vi "Data Type to I32.vi"(8 "error in (no error)":errorcluster, 11 "Data Type":refnum<class "Data Type.lvclass">) -> (0 "error out":errorcluster, 3 "I32 out":i32)   [LabVIEW 2017, in "I32.lvclass"]
uses:
  <vilib>/gpm_packages/@cs/data-type-serializer/source/I32/I32.lvclass
  <vilib>/gpm_packages/@cs/data-type-serializer/source/Data Type/Data Type.lvclass
  <vilib>/gpm_packages/@cs/data-type-serializer/source/I32/I32.lvclass/I32.ctl
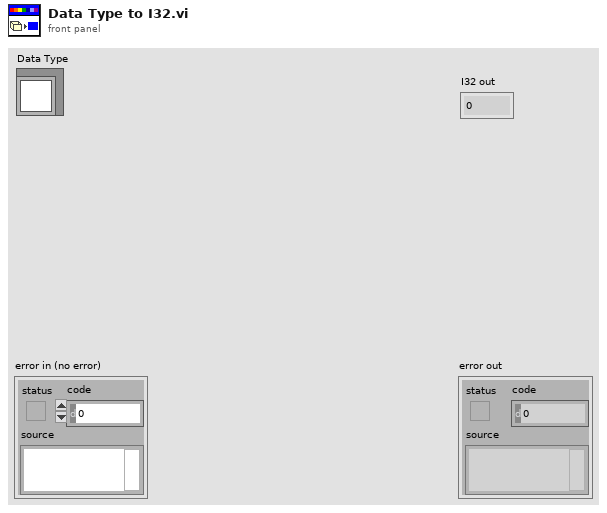
[diagram p1: front panel]
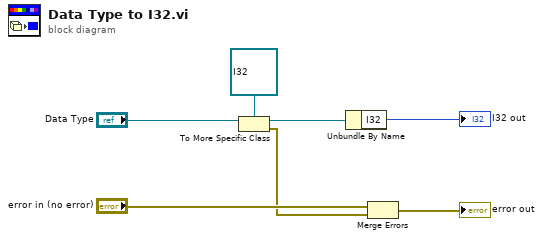
[diagram p0: block diagram]
diagram:
  n1 = To More Specific Class(target class=refnum<class "I32.lvclass"> refnum ("Boolean out"), reference="Data Type") -> (specific class reference=w4:refnum<class "I32.lvclass">, error out=w1:errorcluster)  [unwired: 1 in]
  n2 = Unbundle By Name(w4) -> ("I32"=→"I32 out":i32)
  n3 = Merge Errors("error in (no error)", w1) -> (→"error out":errorcluster)
